vi "DHE_GetModRef_bak.vi"() -> (7 "DHE_ModRef":refnum<vi>)   [LabVIEW 2016]
panel:
  in  "type specifier VI Refnum (for type only)":refnum<vi>
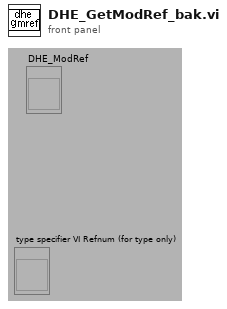
[diagram p1: front panel]
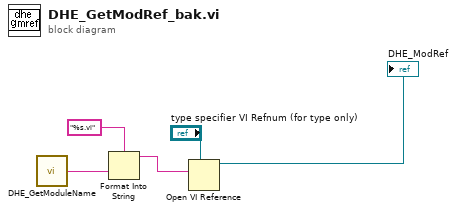
[diagram p0: block diagram]
diagram:
  n1 = call "DHE_GetModuleName.vi"() -> ("DHE_ModuleName"=w3:string)  [unwired: 9 out]
  n2 = Format Into String(format string="%s.vi", w3) -> (resulting string=w2:string)  [unwired: 2 in, 1 out]
  n3 = Open VI Reference(type specifier VI Refnum (for type only)="type specifier VI Refnum (for type only)", vi path=w2) -> (vi reference=→"DHE_ModRef":refnum<vi>)  [unwired: 1 in, 4 out]
